vi "runScript.vi"(6 "data":variant, 8 "error in (no error)":errorcluster, 9 "CompiledList":refnum<class "CompiledList.lvclass">, 10 "HWControllerEvents in":refnum<class "HWControllerEvents.lvclass">, 11 "Compiler in":refnum<class "Compiler.lvclass">) -> (0 "error out":errorcluster, 3 "Compiler out":refnum<class "Compiler.lvclass">)   [LabVIEW 2009, in "Compiler.lvlib" / "Compiler.lvclass"]
uses:
  Compiler.lvclass
  CompiledList/CompiledList.lvclass
  Hal/HWController/HWControllerEvents/HWControllerEvents.lvclass
  Compiler.lvclass/Compiler.ctl
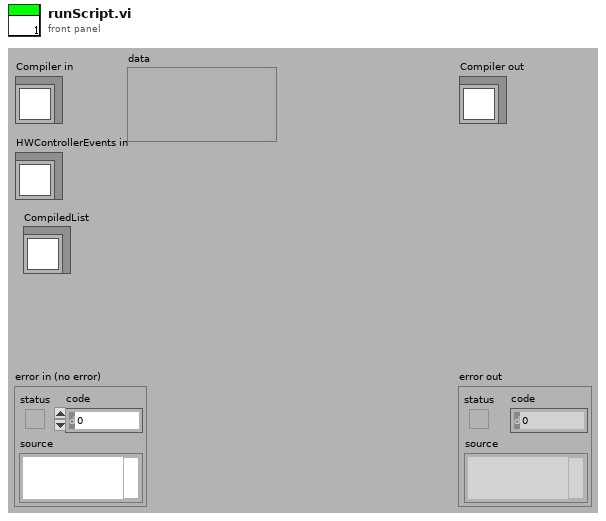
[diagram p1: front panel]
types:
  T1 = enum16{"start", "stop", "statusInquiry", "configure", "resetError", "resourcesInquiry", "reserveResources", "initialise", "resetAllChannels", "staticUpdate", "close", "HWStatus", "error", "resourcesAvailable", "resourcesReserved", "compilerError", "compiledScript", "compilingScript", "runScript", "configureCompiledScript"}
  T2 = cluster{"incomingEventTypes":cluster{"start":cluster{"Boolean":bool}, "stop":cluster{"Boolean":bool}, "statusInquiry":cluster{"Boolean":bool}, "configure":cluster{"DPScriptPath":path, "TimeStamp":string, "HWLoop?":bool}, "resetError":cluster{"Boolean":bool}, "resourcesInquiry":cluster{"Boolean":bool}, "reserveResources":cluster{"HWList":string[]}, "initialise":cluster{"HWList":string[]}, "close":cluster{"Boolean":bool}, "resetAllChannels":cluster{"Boolean":bool}, "staticChannelUpdate":cluster{"channel_address":string, "calibratedValue":dbl}, "runScript":cluster{"DPScriptPath":path, "TimeStamp":string, "HWLoop?":bool}, "compilingScript":cluster{"Path":path}, "compiledScript":cluster{"Path":path, "timeCompileAt":string}, "compilerError":cluster{"Path":path}, "configureCompiledScript":cluster{"DPScriptPath":path, "TimeStamp":string, "HWLoop?":bool, "CompiledScript":cluster{"ScriptListCompiler.lvclass":refnum<class "ScriptListCompiler.lvclass">, "aoChannels":refnum<class "AnalogOutput.lvclass">[], "doChannels":refnum<class "DigitalOutput.lvclass">[], "rfChannels":refnum<class "DDSOutput.lvclass">[]}}, "restartCompiler":cluster{"restart":bool}, "staticRfChannelUpdate":cluster{"channel_address":string, "Output":cluster{"Frequency(MHz)":dbl, "Amplitude":dbl, "Phase":dbl, "OutputForm":enum16{"Sine", "Square", "Triangle", "Arbitrary"}}}, "cameraUpdate":cluster{"Camera":string, "Type":string, "settings":path}}, "outgoingEventTypes":cluster{"HWStatus":cluster{"status":enum16{"Ready", "Compiling", "Configured", "Running", "Stopping", "Unresolved Error"}}, "error":cluster{"error out":errorcluster}, "resourcesAvailable":cluster{"availableHWList":string[], "reservedHWList":string[]}, "resourcesReserved":cluster{"reservedHWList":string[]}}}
  T3 = cluster{"DPScriptPath":path, "TimeStamp":string, "HWLoop?":bool, "CompiledScript":cluster{"ScriptListCompiler.lvclass":refnum<class "ScriptListCompiler.lvclass">, "aoChannels":refnum<class "AnalogOutput.lvclass">[], "doChannels":refnum<class "DigitalOutput.lvclass">[], "rfChannels":refnum<class "DDSOutput.lvclass">[]}}
  T4 = cluster{"DPScriptPath":path, "TimeStamp":string, "HWLoop?":bool}
  T5 = cluster{"ScriptListCompiler.lvclass":refnum<class "ScriptListCompiler.lvclass">, "aoChannels":refnum<class "AnalogOutput.lvclass">[], "doChannels":refnum<class "DigitalOutput.lvclass">[], "rfChannels":refnum<class "DDSOutput.lvclass">[]}
  T6 = cluster{"eventId":enum16{"start", "stop", "statusInquiry", "configure", "resetError", "resourcesInquiry", "reserveResources", "initialise", "resetAllChannels", "staticUpdate", "close", "HWStatus", "error", "resourcesAvailable", "resourcesReserved", "compilerError", "compiledScript", "compilingScript", "runScript", "configureCompiledScript"}, "configureCompiledScript":cluster{"DPScriptPath":path, "TimeStamp":string, "HWLoop?":bool, "CompiledScript":cluster{"ScriptListCompiler.lvclass":refnum<class "ScriptListCompiler.lvclass">, "aoChannels":refnum<class "AnalogOutput.lvclass">[], "doChannels":refnum<class "DigitalOutput.lvclass">[], "rfChannels":refnum<class "DDSOutput.lvclass">[]}}}
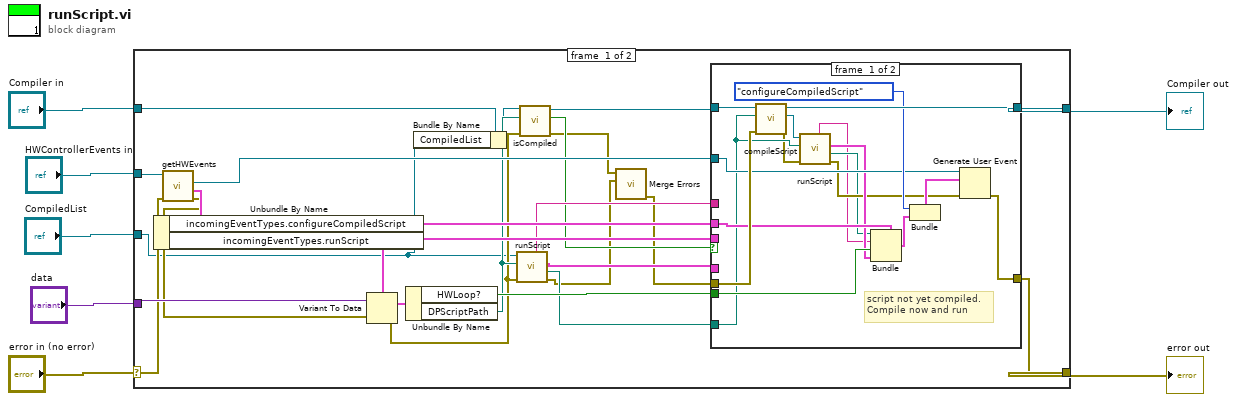
[diagram p0: block diagram]
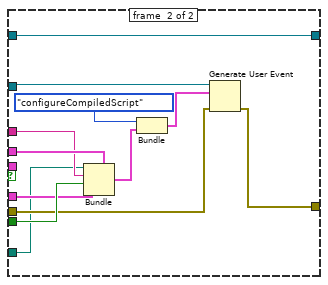
[diagram p2: hidden frame]
diagram:
  n1 = case shown="No Error" "error in (no error)" {
    selector: "error in (no error)" -> [w22 w63]
    tunnel: [w25 w63] -> w6
    tunnel: [w28 w62] -> w4
    tunnel: "Compiler in" -> [w9 w62]
    tunnel: "HWControllerEvents in" -> [w32 _]
    tunnel: "CompiledList" -> [w10 _]
    tunnel: "data" -> [w30 _]
    frame #0 {
      n2 = call-dynamic "getHWEvents.vi"("error in (no error)"=w22, "HWControllerEvents in"=w32) -> ("error out"=w21:errorcluster, "eventDataTypes"=w31:T2, "HWCEvent"=w26:refnum<user-event>)  [unwired: 6 in, 1 out]
      n3 = Unbundle By Name(w31) -> ("incomingEventTypes.configureCompiledScript"=w24:T3, "incomingEventTypes.runScript"=w23:T4)
      n4 = Variant To Data(error in=w21, Variant=w30, type=w23) -> (error out=w16:errorcluster, data=w29:T4)
      n5 = Unbundle By Name(w29) -> ("HWLoop?"=w27:bool, "DPScriptPath"=w17:path)
      n6 = Bundle By Name(cluster=w9, "CompiledList"=w10) -> (w8:refnum<class "Compiler.lvclass">)
      n7 = call "runScript.vi"("error in (no error)"=w16, "Path"=w17, "CompiledList in"=w10) -> ("error out"=w12:errorcluster, "Path out"=w19:path, "CompiledScript"=w20:T5, "TimeStamp"=w18:string)  [unwired: 3 in, 2 out]
      n8 = call "isCompiled.vi"("error in (no error)"=w16, "Path"=w17, "Compiler in"=w8) -> ("error out"=w13:errorcluster, "compiled?"=w15:bool, "Compiler out"=w14:refnum<class "Compiler.lvclass">)  [unwired: 6 in]
      n9 = call <vilib>:"Merge Errors.vi"("error in 2 (no error)"=w12, "error in 1 (no error)"=w13) -> ("error out"=w11:errorcluster)  [unwired: 5 in]
      n10 = case shown="True" w15 {
        tunnel: w20 -> [_ w58]
        tunnel: [w48 w61] -> w28
        tunnel: w14 -> [w49 w61]
        tunnel: w11 -> [w47 w53]
        tunnel: w27 -> [w42 w59]
        tunnel: w26 -> [w40 w57]
        tunnel: [w41 w52] -> w25
        tunnel: w24 -> [w43 w60]
        tunnel: w19 -> [w38 w50]
        tunnel: w23 -> [_ _]
        tunnel: w18 -> [_ w51]
        frame #0 {
          # "script not yet compiled.\nCompile now and run"
          n11 = call "compileScript.vi"("error in (no error)"=w47, "Path"=w38, "Compiler in"=w49) -> ("error out"=w37:errorcluster, "CompiledList"=w39:refnum<class "CompiledList.lvclass">, "Compiler out"=w48:refnum<class "Compiler.lvclass">)  [unwired: 6 in]
          n12 = call "runScript.vi"("error in (no error)"=w37, "Path"=w38, "CompiledList in"=w39) -> ("error out"=w35:errorcluster, "Path out"=w34:path, "CompiledScript"=w36:T5, "TimeStamp"=w33:string)  [unwired: 3 in, 2 out]
          n13 = Bundle(cluster=w43, "DPScriptPath"=w34, "TimeStamp"=w33, "HWLoop?"=w42, "CompiledScript"=w36) -> (w45:T3)
          n14 = Bundle("eventId"=T1."configureCompiledScript", "configureCompiledScript"=w45) -> (w44:T6)  [unwired: 1 in]
          n15 = Generate User Event(user event=w40, event data cluster=w44, error in=w35) -> (error out=w41:errorcluster)  [unwired: 1 out]
        }
        frame #1 {
          n16 = Bundle(cluster=w60, "DPScriptPath"=w50, "TimeStamp"=w51, "HWLoop?"=w59, "CompiledScript"=w58) -> (w55:T3)
          n17 = Bundle("eventId"=T1."configureCompiledScript", "configureCompiledScript"=w55) -> (w54:T6)  [unwired: 1 in]
          n18 = Generate User Event(user event=w57, event data cluster=w54, error in=w53) -> (error out=w52:errorcluster)  [unwired: 1 out]
        }
      }
    }
    frame #1 {
    }
  }
  "error out" <- w6
  "Compiler out" <- w4
